vi "MSTDaily.vi"() -> ()   [LabVIEW 2012]
uses:
  <vilib>/addons/database/Connection.llb/DB Tools Open Connec (Path).vi
  <vilib>/addons/database/Connection.llb/Conn Execute.vi
  <vilib>/addons/database/Recordset.llb/Rec Fetch Recordset Data (R).vi
  <vilib>/addons/database/Recordset.llb/Rec Destroy - Connection.vi
  <vilib>/addons/database/_DB Variant To Data/Database Variant To Data.xnode
  <vilib>/addons/database/NI_Database_API.lvlib
  <vilib>/Utility/NIReport.llb/Excel/NI_Excel.lvclass
  <vilib>/Utility/NIReport.llb/NI_report.lvclass
panel:
  out "error out":errorcluster
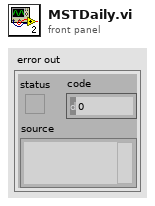
[diagram p1: front panel]
types:
  T1 = enum16{"Standard Report", "HTML", "Word", "Excel"}
  T2 = typedef "NI_Database_API.lvlib/Conn ObjectReference.ctl" = refnum<k1>
  T3 = typedef "NI_Database_API.lvlib/Rec ObjectReference.ctl" = refnum<k1>
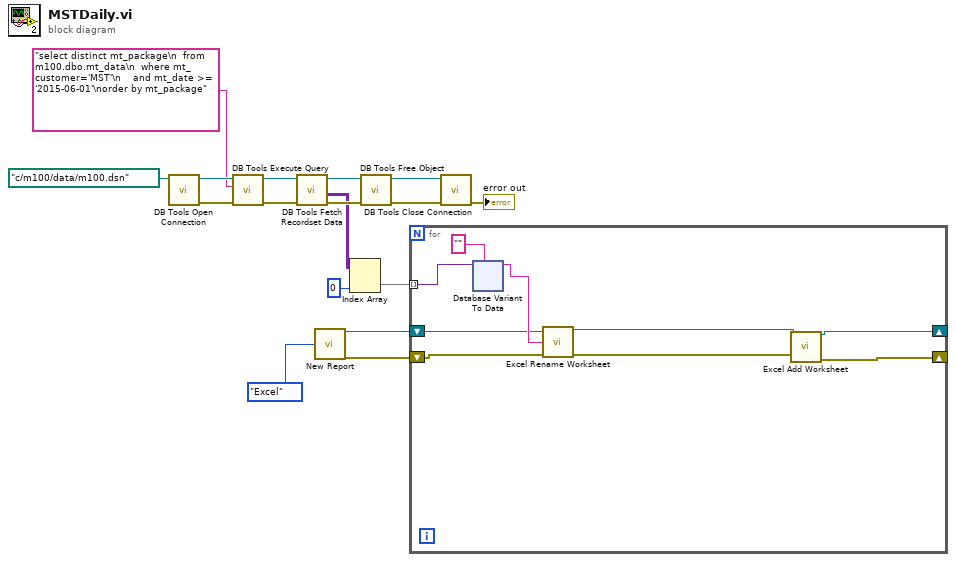
[diagram p0: block diagram]
diagram:
  n1 = call-poly <vilib>:"DB Tools Open Connection.vi"("connection information"=path "c:/m100/data/m100.dsn") -> ("error out"=w12:errorcluster, "connection reference"=w14:T2)  [unwired: 7 in]
  n2 = call-poly <vilib>:"DB Tools Execute Query.vi"("error in (no error)"=w12, "SQL query"="select distinct mt_package\n  from m100.dbo.mt_data\n  where mt_customer='MST'\n    and mt_date >= '2015-06-01'\norder by mt_package", "connection reference"=w14) -> ("error out"=w11:errorcluster, "recordset reference"=w17:T3)  [unwired: 5 in]
  n3 = call-poly <vilib>:"DB Tools Fetch Recordset Data.vi"("error in (no error)"=w11, "recordset reference"=w17) -> ("error out"=w10:errorcluster, "recordset data"=w6:variant[][], "recordset reference out"=w16:T3)  [unwired: 3 in]
  n4 = call <vilib>:"New Report.vi"("report type"=T1."Excel") -> ("report out"=w2:refnum<class "NI_report.lvclass">, "error out"=w1:errorcluster)  [unwired: 13 in]
  n5 = Index Array(array=w6, index (col)=0 ("disabled index (col)")) -> (element=w4:variant[])  [unwired: 1 in]
  n6 = call-poly <vilib>:"DB Tools Free Object.vi"("error in (no error)"=w10, "recordset reference"=w16) -> ("error out"=w9:errorcluster, "connection reference"=w15:T2)  [unwired: 8 in]
  n7 = for {
    tunnel: w4 -> [w26] mode=indexing
    shift-right: [w21] -> _
    shift-left: w2 -> [w19]
    shift-right: [w20] -> _
    shift-left: w1 -> [w18]
    n8 = xnode "Database Variant To Data"("database variant"=w26, "type"="") -> ("data"=w24:string)  [unwired: 1 in, 1 out]
    n9 = call <vilib>:"Excel Rename Worksheet.vi"("report in"=w19, "worksheet name (\"\")"=w24, "error in (no error)"=w18) -> ("report out"=w23:refnum<class "NI_report.lvclass">, "error out"=w22:errorcluster)  [unwired: 11 in]
    n10 = call <vilib>:"Excel Add Worksheet.vi"("report in"=w23, "error in (no error)"=w22) -> ("report out"=w21:refnum<class "NI_report.lvclass">, "error out"=w20:errorcluster)  [unwired: 12 in]
  }
  n11 = call <vilib>:"DB Tools Close Connection.vi"("error in (no error)"=w9, "connection reference"=w15) -> ("error out"=→"error out":errorcluster)  [unwired: 5 in]
